vi "Do.vi"(8 "error in (no error)":errorcluster, 10 "Counter In":refnum<class "Counter.lvclass">, 11 "Stop in":refnum<class "Stop.lvclass">) -> (0 "error out":errorcluster, 2 "Counter Out":refnum<class "Counter.lvclass">, 3 "Stop out":refnum<class "Stop.lvclass">)   [LabVIEW 2018, in "Stop.lvclass"]
uses:
  Stop.lvclass
  Counter Class/Counter.lvclass
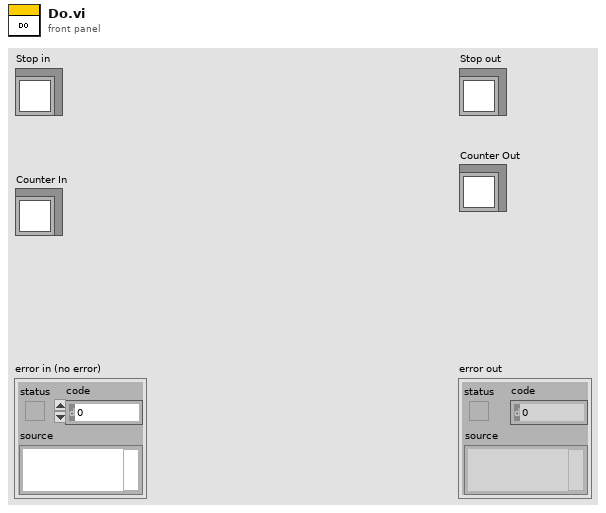
[diagram p1: front panel]
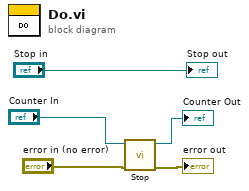
[diagram p0: block diagram]
diagram:
  n1 = call-dynamic "Stop.vi"("error in (no error)"="error in (no error)", "Counter in"="Counter In") -> ("error out"=→"error out":errorcluster, "Counter out"=→"Counter Out":refnum<class "Counter.lvclass">)  [unwired: 8 in]
  "Stop out" <- "Stop in"
